vi "Debouncer_Calculate.vi"(8 "CurrentTIme":dbl=-1.0, 10 "Input":bool, 11 "Debouncer In":T1 {"PrevTimeSeconds" format="%13.6p"; "DebounceTimeSeconds" format="%13.6p"}) -> (0 "CurrentTIme Out":dbl, 2 "Output":bool, 3 "Debouncer Out":T1 {"PrevTimeSeconds" format="%13.6p"; "DebounceTimeSeconds" format="%13.6p"})   [LabVIEW 2019, in "Trajectory_Library.lvlib"]
doc: "Applies the debouncer to the input stream.\n\nInputs:\n - DebounceIn -- Debounce data cluster\n - input -- The current value of the input stream.\n - CurrentTime -- (Optional - Default: read system timer) The current system elapsed time.\n\nOutputs:\n - DebouceOut -- Updated data cluster\n - output -- The debounced value of the input stream.\n - CurrentTimeOut -- The current system time. If not read and not supplied, value will be -1.0."
uses:
  Trajectory_Library.lvlib
  Enum/DEBOUNCER_TYPE_ENUM.ctl
  TypeDef/DEBOUNCER.ctl
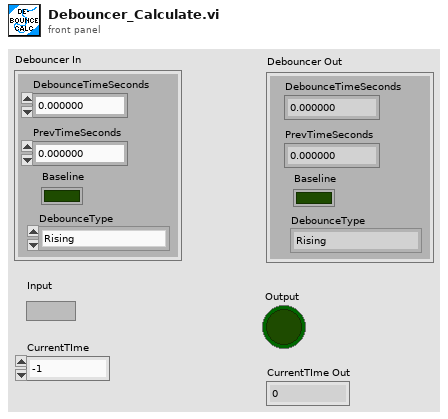
[diagram p1: front panel]
types:
  T1 = typedef "Trajectory_Library.lvlib/DEBOUNCER.ctl" = cluster{"DebounceTimeSeconds":dbl, "PrevTimeSeconds":dbl, "Baseline":bool, "DebounceType":T2}
  T2 = typedef "Trajectory_Library.lvlib/DEBOUNCER_TYPE_ENUM.ctl" = enum16{"Rising", "Falling", "Both"}
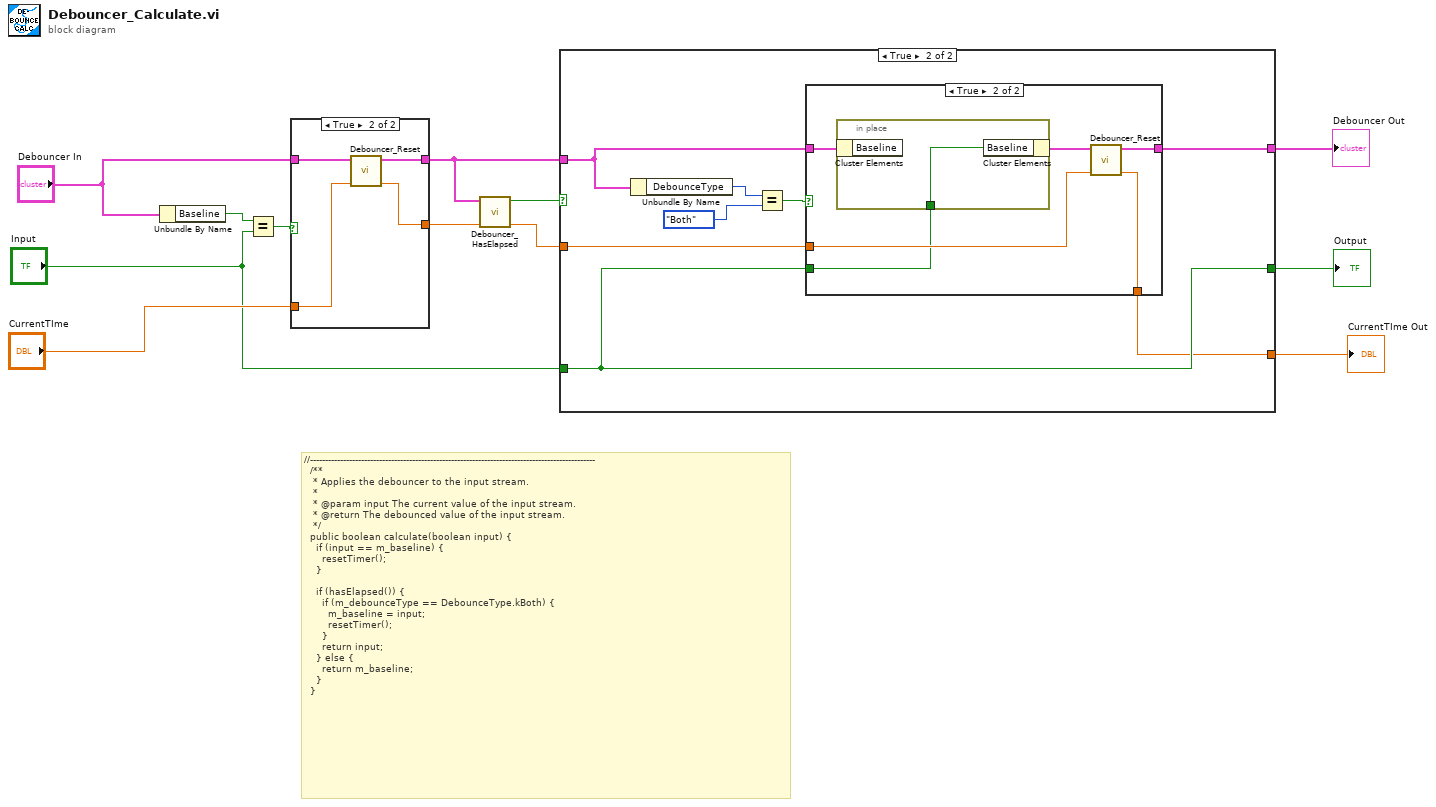
[diagram p0: block diagram]
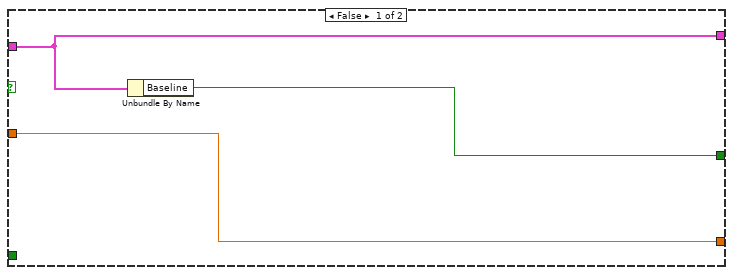
[diagram p2: hidden frame]
diagram:
  # "//-----------------------------------------------------------------------------------------------\n  /**\n   * Applies the debouncer to the input stream.\n   *\n   * @param input The current value of the input stream.\n   * @return The debounced value of the input stream.\n   */\n  public boolean calculate(boolean input) {\n    if (input == m_baseline) {\n      resetTimer();\n    }\n\n    if (hasElapsed()) {\n      if (m_debounceType == DebounceType.kBoth) {\n        m_baseline = input;\n        resetTimer();\n      }\n      return input;\n    } else {\n      return m_baseline;\n    }\n  }"
  n1 = Unbundle By Name("Debouncer In") -> ("Baseline"=w12:bool)
  n2 = Equal?(x=w12, y="Input") -> (x = y?=w11:bool)
  n3 = case shown="True" w11 {
    tunnel: "Debouncer In" -> [w14 w18]
    tunnel: "CurrentTIme" -> [w13 w16]
    tunnel: [w14 w17] -> w6
    tunnel: [w13 w15] -> w8
    frame False {
    }
    frame True {
      n4 = call "Debouncer_Reset.vi"("CurrentTIme"=w16, "Debouncer In"=w18) -> ("CurrentTIme Out"=w15:dbl, "Debouncer Out"=w17:T1)  [unwired: 8 in]
    }
  }
  n5 = call "Debouncer_HasElapsed.vi"("CurrentTIme"=w8, "Debouncer In"=w6) -> ("CurrentTimeOut"=w4:dbl, "HasElapsed"=w7:bool)  [unwired: 8 in]
  n6 = case shown="True" w7 {
    tunnel: w6 -> [w20 w26]
    tunnel: "Input" -> [_ w24]
    tunnel: w4 -> [w19 w25]
    tunnel: [w21 w24] -> w3
    tunnel: [w20 w23] -> w2
    tunnel: [w19 w22] -> w1
    frame False {
      n7 = Unbundle By Name(w20) -> ("Baseline"=w21:bool)
    }
    frame True {
      n8 = Unbundle By Name(w26) -> ("DebounceType"=w29:T2)
      n9 = Equal?(x=w29, y=DEBOUNCER_TYPE_ENUM."Both") -> (x = y?=w27:bool)
      n10 = case shown="True" w27 {
        tunnel: w26 -> [w31 w37]
        tunnel: w24 -> [_ w34]
        tunnel: w25 -> [w30 w35]
        tunnel: [w31 w33] -> w23
        tunnel: [w30 w32] -> w22
        frame False {
        }
        frame True {
          n11 = in-place {
            in-place-border: w34 -> [w38]
            n12 = in-place-cluster #1(w37) -> ()  [unwired: 1 out]
            n13 = in-place-cluster #1("Baseline"=w38) -> (w36:T1)
          }
          n14 = call "Debouncer_Reset.vi"("CurrentTIme"=w35, "Debouncer In"=w36) -> ("CurrentTIme Out"=w32:dbl, "Debouncer Out"=w33:T1)  [unwired: 8 in]
        }
      }
    }
  }
  "Debouncer Out" <- w2
  "Output" <- w3
  "CurrentTIme Out" <- w1
